vi "Load Boot-up Profile.vi"(8 "error in (no error)":errorcluster, 11 "Controller in":refnum<class "Controller.lvclass">) -> (0 "error out":errorcluster, 2 "data":T1, 3 "Controller out":refnum<class "Controller.lvclass">)   [LabVIEW 2016, in "Controller Actor.lvlib" / "Controller.lvclass"]
uses:
  <userlib>/Common Components/Controller/Controller.lvclass
  <userlib>/Common Components/Controller/Controller.lvclass/Controller.ctl
  <vilib>/Utility/config.llb/NI_LVConfig.lvlib
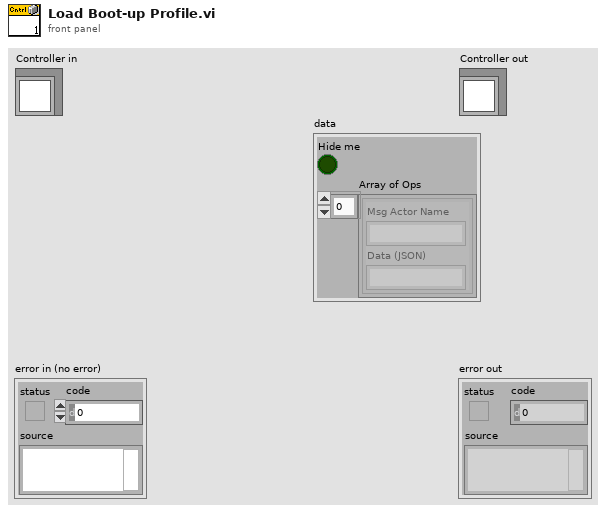
[diagram p1: front panel]
types:
  T1 = cluster{"Hide me":bool, "Array of Ops":cluster{"Msg Actor Name":string, "Data (JSON)":string}[]}
  T2 = typedef "NI_LVConfig.lvlib/Config Data RefNum.ctl" = refnum<k1>
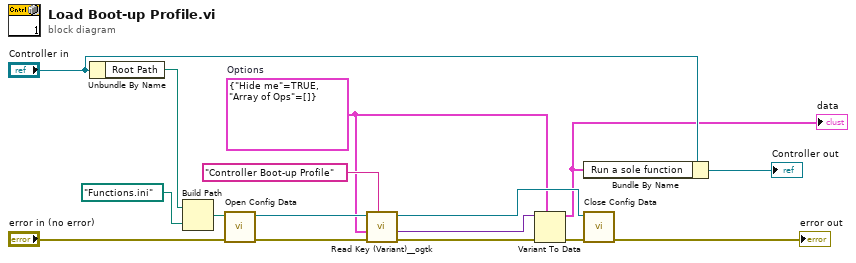
[diagram p0: block diagram]
diagram:
  w9 = T1 {"Hide me"=TRUE, "Array of Ops"=[]}  # Options
  n1 = Unbundle By Name("Controller in") -> ("Root Path"=w5:path)
  n2 = Build Path(base path=w5, name or relative path=path "Functions.ini" ("VI Path")) -> (appended path=w3:path)
  n3 = call <vilib>:"Open Config Data.vi"("error in (no error)"="error in (no error)", "configuration file path"=w3) -> ("error out"=w12:errorcluster, "refnum"=w16:T2)  [unwired: 7 in, 1 out]
  n4 = call <userlib>:"Read Key (Variant)__ogtk.vi"("section"="Controller Boot-up Profile", "error in (no error)"=w12, "type"=w9, "refnum"=w16) -> ("error out"=w11:errorcluster, "key-value"=w13:variant, "refnum out"=w15:T2)  [unwired: 4 in, 1 out]
  n5 = Variant To Data(error in=w11, type=w9, Variant=w13) -> (data=w1:T1, error out=w10:errorcluster)
  "data" <- w1
  n6 = Bundle By Name(cluster="Controller in", "Run a sole function"=w1) -> (→"Controller out":refnum<class "Controller.lvclass">)
  n7 = call <vilib>:"Close Config Data.vi"("error in (no error)"=w10, "refnum"=w15) -> ("error out"=→"error out":errorcluster)  [unwired: 8 in, 1 out]
